vi "EdgePointUnderMouse.vi"(0 "FSM.Graph In":refnum<class "FSM.Graph.lvclass">, 7 "Coords":T1) -> (4 "FSM.Graph Out":refnum<class "FSM.Graph.lvclass">, 15 "edge point?":bool)   [LabVIEW 2020, in "FSM.Graph.lvclass"]
uses:
  FSM.Graph.lvclass
  <vilib>/Utility/miscctls.llb/LVPoint32TypeDef.ctl
  FSM.Graph.lvclass/FSM.Graph.ctl
  FSM.Edge/FSM.Edge.lvclass
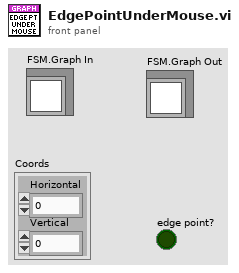
[diagram p1: front panel]
types:
  T1 = typedef "LVPoint32TypeDef.ctl" = cluster{"Horizontal":i32, "Vertical":i32}
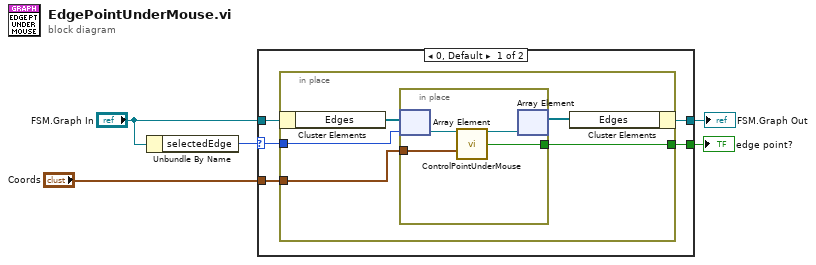
[diagram p0: block diagram]
diagram:
  n1 = Unbundle By Name("FSM.Graph In") -> ("selectedEdge"=w4:i32)
  n2 = case shown="0, Default" w4 {
    selector: w4 -> [w6 _]
    tunnel: "Coords" -> [w10 _]
    tunnel: [w9 _] -> w3
    tunnel: "FSM.Graph In" -> [w8 w20]
    tunnel: [w7 w20] -> w1
    frame 0, Default {
      n3 = in-place {
        in-place-border: w10 -> [w15]
        in-place-border: [w14] -> w9
        in-place-border: w6 -> [w11]
        n4 = in-place-cluster #1(w8) -> ("Edges"=w13:refnum<class "FSM.Edge.lvclass">[])
        n5 = in-place {
          in-place-border: w15 -> [w19]
          in-place-border: [w18] -> w14
          n6 = in-place-array #2(w13, w11) -> (w16:refnum<class "FSM.Edge.lvclass">)
          n7 = call "ControlPointUnderMouse.vi"("FSM.Edge In"=w16, "Coords"=w19) -> ("FSM.Edge Out"=w17:refnum<class "FSM.Edge.lvclass">, "control point?"=w18:bool)  [unwired: 11 in, 1 out]
          n8 = in-place-array #2(w17) -> (w12:refnum<class "FSM.Edge.lvclass">[])  [unwired: 1 out]
        }
        n9 = in-place-cluster #1("Edges"=w12) -> (w7:refnum<class "FSM.Graph.lvclass">)
      }
    }
    frame -1 {
    }
  }
  "FSM.Graph Out" <- w1
  "edge point?" <- w3
